vi "数据记录.vi"(11 "写入字段":string) -> (3 "连接的字符串":string)   [LabVIEW 2016]
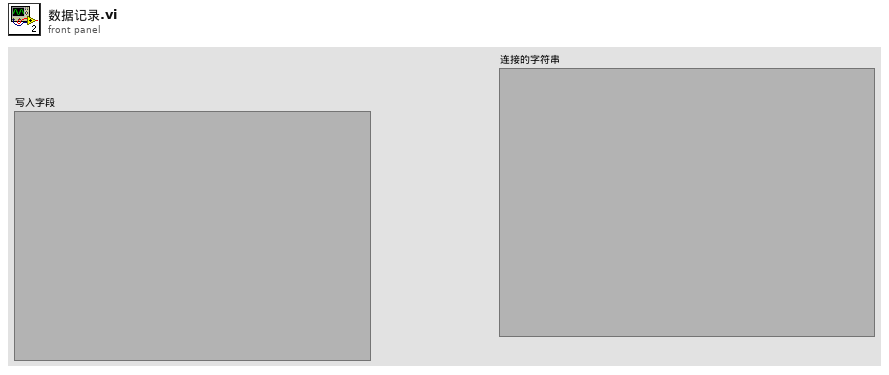
[diagram p1: front panel]
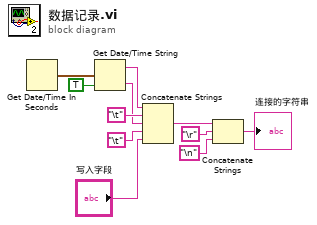
[diagram p0: block diagram]
diagram:
  n1 = Get Date/Time In Seconds() -> (seconds since 1Jan1904=w3:timestamp)
  n2 = Get Date/Time String(seconds (now)=w3, want seconds? (F)=TRUE ("需要秒？(F)")) -> (date string=w6:string, time string=w4:string)  [unwired: 1 in]
  n3 = Concatenate Strings(w6, "\t", w4, "\t", "写入字段") -> (w1:string)
  n4 = Concatenate Strings(w1, "\r", "\n") -> (→"连接的字符串":string)
